vi "Q8381 Header Judge.vi"(0 "String":string) -> (1 "Judge":string, 2 "Output":bool)   [LabVIEW 2017]
doc: "Judge if there exists header or not by checking if there is any +, - or (space) at third or fifth digit. If input string includes header output = T."
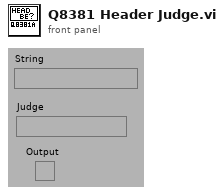
[diagram p1: front panel]
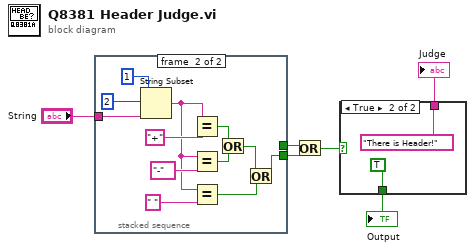
[diagram p0: block diagram]
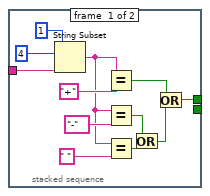
[diagram p2: hidden frame]
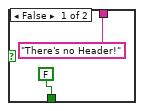
[diagram p3: hidden frame]
diagram:
  n1 = stacked-sequence {
    tunnel: "String" -> [w11 w19]
    tunnel: [w7 _] -> w3
    tunnel: [_ w20] -> w2
    frame #0 {
      n2 = String Subset(string=w11, offset (0)=4, length (rest)=1) -> (substring=w16:string)
      n3 = Equal?(x=w16, y="+") -> (x = y?=w14:bool)
      n4 = Equal?(x=w16, y="-") -> (x = y?=w9:bool)
      n5 = Equal?(x=w16, y=" ") -> (x = y?=w10:bool)
      n6 = Or(x=w9, y=w10) -> (x .or. y?=w8:bool)
      n7 = Or(x=w14, y=w8) -> (x .or. y?=w7:bool)
    }
    frame #1 {
      n8 = String Subset(string=w19, offset (0)=2, length (rest)=1) -> (substring=w28:string)
      n9 = Equal?(x=w28, y="+") -> (x = y?=w26:bool)
      n10 = Equal?(x=w28, y="-") -> (x = y?=w25:bool)
      n11 = Equal?(x=w28, y=" ") -> (x = y?=w23:bool)
      n12 = Or(x=w26, y=w25) -> (x .or. y?=w24:bool)
      n13 = Or(x=w24, y=w23) -> (x .or. y?=w20:bool)
    }
  }
  n14 = Or(x=w3, y=w2) -> (x .or. y?=w1:bool)
  n15 = case shown="True" w1 {
    tunnel: [FALSE TRUE] -> w5
    tunnel: ["There's no Header!" "There is Header!"] -> w6
    frame False {
    }
    frame True {
    }
  }
  "Judge" <- w6
  "Output" <- w5
